vi "Test Get ATM Message on Inquiry Account Balance After Database Update.vi"(8 "error in (no error)":errorcluster, 11 "Test Case In":refnum<class "Controller Test.lvclass">) -> (0 "error out":errorcluster, 3 "Test Case Out":refnum<class "Controller Test.lvclass">)   [LabVIEW 2020, in "Controller Test.lvclass"]
uses:
  Controller Test/Controller Test.lvclass
  Controller Test/Controller Test.lvclass/Controller Test.ctl
  01074fa8-ee8a-411d-bc8b-fc92c4f90959.vi
  ATM Controller/ATM Controller.lvclass
  Account Database/Account Data.ctl
  Account Database/Account Database.lvclass
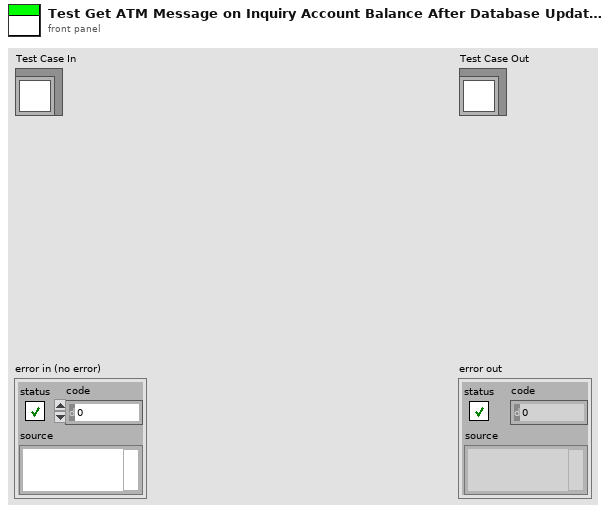
[diagram p1: front panel]
types:
  T1 = typedef "Account Database.lvclass/Account Data.ctl" = cluster{"Account Number":string, "First Name":string, "Last Name":string, "Account Balance":string}
  T2 = typedef "ATM Controller.lvclass/State.ctl" = enum16{"Start", "Card Inserted", "Verification Failed", "Verification Succeeded", "Depositing", "Depositing Completed", "Withdrawing", "Withdraw Completed", "Withdraw Failed", "Balance Inquiry", "Terminate"}
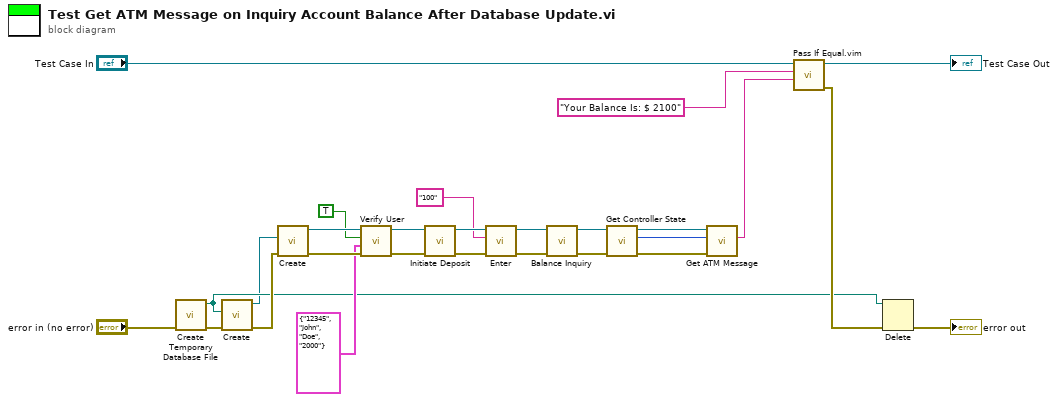
[diagram p0: block diagram]
diagram:
  n1 = call "Create Temporary Database File.vi"("error in (no error)"="error in (no error)") -> ("error out"=w11:errorcluster, "path"=w8:path)  [unwired: 9 in]
  n2 = call "Create.vi"("error in (no error)"=w11, "Data File"=w8) -> ("error out"=w10:errorcluster, "Account Database out"=w7:refnum<class "Account Database.lvclass">)  [unwired: 8 in]
  n3 = call "Create.vi"("error in (no error)"=w10, "Account Database"=w7) -> ("error out"=w23:errorcluster, "ATM Controller out"=w21:refnum<class "ATM Controller.lvclass">)  [unwired: 8 in]
  n4 = call "Verify User.vi"("error in (no error)"=w23, "Account Data"=T1 {"Account Number"="12345", "First Name"="John", "Last Name"="Doe", "Account Balance"="2000"}, "Verified?"=TRUE, "ATM Controller in"=w21) -> ("error out"=w22:errorcluster, "ATM Controller out"=w5:refnum<class "ATM Controller.lvclass">)  [unwired: 6 in]
  n5 = call "Initiate Deposit.vi"("error in (no error)"=w22, "ATM Controller in"=w5) -> ("error out"=w6:errorcluster, "ATM Controller out"=w3:refnum<class "ATM Controller.lvclass">)  [unwired: 8 in]
  n6 = call "Enter.vi"("error in (no error)"=w6, "User Input"="100", "ATM Controller in"=w3) -> ("error out"=w4:errorcluster, "ATM Controller out"=w2:refnum<class "ATM Controller.lvclass">)  [unwired: 7 in]
  n7 = call "Balance Inquiry.vi"("error in (no error)"=w4, "ATM Controller in"=w2) -> ("error out"=w18:errorcluster, "ATM Controller out"=w17:refnum<class "ATM Controller.lvclass">)  [unwired: 8 in]
  n8 = call "Get Controller State.vi"("error in (no error)"=w18, "ATM Controller in"=w17) -> ("error out"=w14:errorcluster, "ATM State"=w15:T2, "ATM Controller out"=w16:refnum<class "ATM Controller.lvclass">)  [unwired: 7 in]
  n9 = call "Get ATM Message.vi"("error in (no error)"=w14, "ATM State"=w15, "ATM Controller In"=w16) -> ("Message"=w13:string)  [unwired: 6 in, 2 out]
  n10 = call "Pass If Equal.vim"("Actual"=w13, "Expected"="Your Balance Is: $ 2100" ("Message"), "LUnit Test Case In"="Test Case In") -> ("error out"=w25:errorcluster, "LUnit Test Case Out"=→"Test Case Out":refnum<class "Controller Test.lvclass">)  [unwired: 7 in]
  n11 = Delete(path (use dialog)=w8, error in=w25) -> (error out=→"error out":errorcluster)  [unwired: 3 in, 2 out]
